vi "Frame Save Loop.vi"(8 "error in (no error)":errorcluster, 11 "SB App in":refnum<class "SB App.lvclass">) -> (0 "error out":errorcluster)   [LabVIEW 2020, in "SB App.lvlib" / "SB App.lvclass"]
uses:
  SB App.lvclass
  SB App.lvclass/SB App.ctl
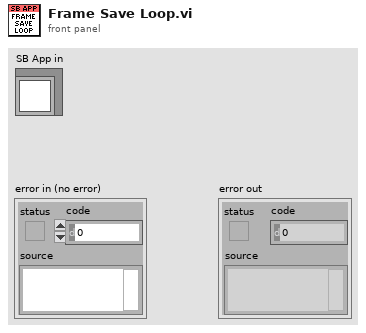
[diagram p1: front panel]
types:
  T1 = typedef "SB App.lvlib/SB App.lvclass/Video Frame.ctl" = cluster{"Image":T2, "Frame Path":path}
  T2 = typedef "imagedata.ctl" = cluster{"image type":i32, "image depth":i32, "image":u8[], "mask":u8[], "colors":u32[], "Rectangle":cluster{"left":i16, "top":i16, "right":i16, "bottom":i16}}
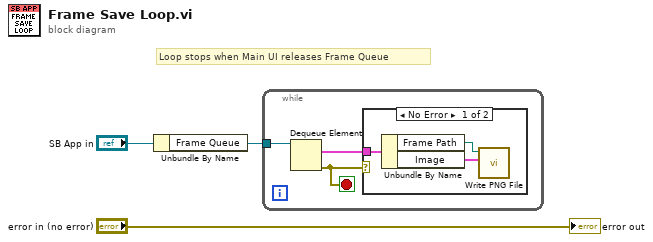
[diagram p0: block diagram]
diagram:
  # "Loop stops when Main UI releases Frame Queue"
  n1 = Unbundle By Name("SB App in") -> ("Frame Queue"=w2:refnum<queue>)
  n2 = while {
    tunnel: w2 -> [w6]
    stop <- w4 stop-if-true
    n3 = Dequeue Element(queue=w6) -> (element=w5:T1, error out=w4:errorcluster)  [unwired: 2 in, 2 out]
    n4 = case shown="No Error" w4 {
      tunnel: w5 -> [w9 _]
      frame No Error {
        n5 = Unbundle By Name(w9) -> ("Frame Path"=w7:path, "Image"=w8:T2)
        n6 = call <vilib>:"Write PNG File.vi"("image data"=w8, "path to PNG file"=w7) -> ()  [unwired: 8 in, 2 out]
      }
      frame Error {
      }
    }
  }
  "error out" <- "error in (no error)"
